vi "Insight_RW_SampleClockRate.vi"(8 "error in (no error)":errorcluster, 9 "Mode (Read / Write)":enum8{"Write", "Read"}(ring), 10 "Clock Rate (MHz)":dbl=400.0, 11 "telnet connection":T1) -> (0 "error out":errorcluster, 1 "response data":string, 2 "Clock Rate (MHz)":dbl, 3 "telnet  connection out":T1)   [LabVIEW 2011]
doc: "Insight Photonic Solutions\n\nThis VI reads or writes the User Sample Clock Rate, in MHz. Use this to change the rate at which data is acquired by an external data acquisition system that is triggered with the laser's Sample Clock output. Be aware that to properly reduce the data with the Data Valid Vector, only use rational dividends of the laser's drive clock (e.g. if drive is 400 MHz, then sample clock rate may be 400/N MHz.)\n\nAlternatively, you are allowed to set the Sample Clock to 10MHz. You may then use the Sample Clock as a Reference Clock to synchronize a data acquisition to, and use the internal data acquisition clock. This mode of operation is experimental.\n\nver 3.2 - original release. Uses this version number, to correlate with older commands that recently incorporate a new parser to handle responses from pre-Atlas 3.1 commands and post version 3.2 commands."
uses:
  Telnet Session.ctl
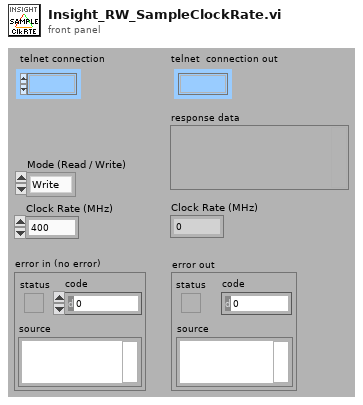
[diagram p1: front panel]
types:
  T1 = typedef "Telnet Session.ctl" = refnum<k1>
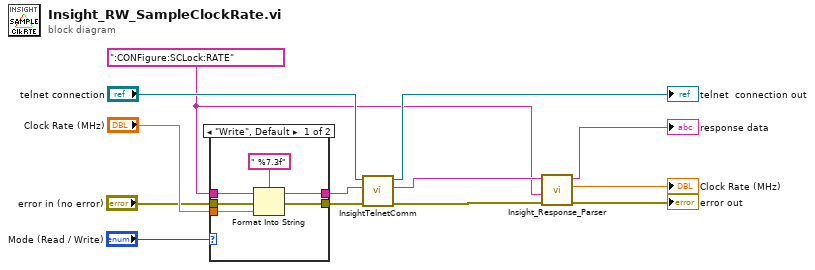
[diagram p0: block diagram]
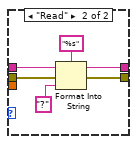
[diagram p2: hidden frame]
diagram:
  w1 = ":CONFigure:SCLock:RATE" ("String")
  n1 = case shown="\"Write\", Default" "Mode (Read / Write)" {
    tunnel: [w19 w21] -> w10
    tunnel: "error in (no error)" -> [w18 w20]
    tunnel: w1 -> [w17 w23]
    tunnel: "Clock Rate (MHz)" -> [w16 _]
    tunnel: [w14 w22] -> w9
    frame "Write", Default {
      n2 = Format Into String(format string=" %7.3f", initial string=w17, error in=w18, w16) -> (resulting string=w14:string, error out=w19:errorcluster)
    }
    frame "Read" {
      n3 = Format Into String(format string="%s", initial string=w23, error in=w20, "?" ("input 1")) -> (resulting string=w22:string, error out=w21:errorcluster)
    }
  }
  n4 = call "InsightTelnetComm.vi"("error in"=w10, "write buffer (\"\")"=w9, "telnet connection"="telnet connection") -> ("error out"=w2:errorcluster, "response data"=w3:string, "telnet  connection out"=→"telnet  connection out":T1)  [unwired: 4 in]
  n5 = call "Insight_Response_Parser.vi"("error in (no error)"=w2, "Command String"=w1, "Laser Response In"=w3) -> ("error out"=→"error out":errorcluster, "Value"=→"Clock Rate (MHz)":dbl, "Laser Response Out"=→"response data":string)  [unwired: 6 in]
